vi "Get DSSS EVM.vi"(8 "error in (no error)":errorcluster, 11 "niDTS WLAN INSTR TX in":refnum<class "niDTS WLAN INSTR TX.lvclass">) -> (0 "error out":errorcluster, 2 "DSSS EVM":T1, 3 "niDTS WLAN INSTR TX out":refnum<class "niDTS WLAN INSTR TX.lvclass">)   [LabVIEW 2015, in "niDTS WLAN.lvlib" / "niDTS WLAN INSTR TX.lvclass"]
uses:
  niDTS WLAN INSTR TX.lvclass
  Tests/Tx Test/Includes/niDTS WLAN Tx Test INC DSSS MOD EVM Results.ctl
  Tests/DSSS Tx Test/Includes/Results/niDTS WLAN DSSS Tx RES EVM ALL.ctl
  Tests/DSSS Tx Test/Includes/Results/niDTS WLAN DSSS Tx RES EVM RMS.ctl
  niDTS WLAN INSTR TX.lvclass/niDTS WLAN INSTR TX.ctl
  RiviInstDriver/niRfsaWlan/Objects/niRfsaWlan.lvclass
  niDTS WLAN.lvlib
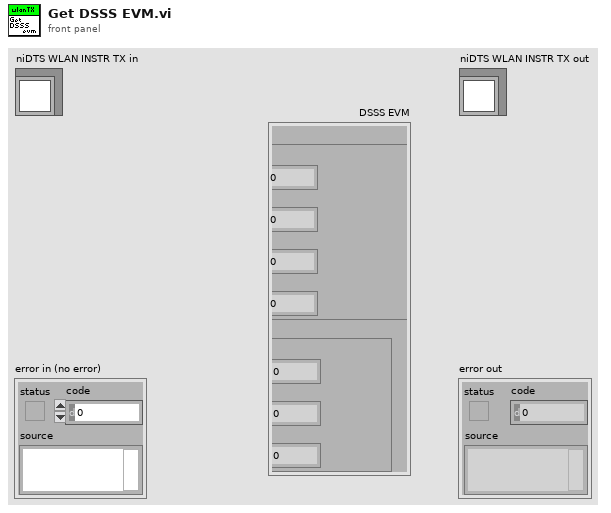
[diagram p1: front panel]
types:
  T1 = typedef "niDTS WLAN.lvlib/niDTS WLAN Tx Test INC DSSS MOD EVM Results.ctl" = cluster{"All":T2, "RMS":T3}
  T2 = typedef "niDTS WLAN.lvlib/niDTS WLAN DSSS Tx RES EVM ALL.ctl" = cluster{"Average RMS EVM (%)":dbl, "Max Peak EVM (%)":dbl, "Max Peak 11b EVM (%)":dbl, "New Max Peak 11b EVM (%)":dbl}
  T3 = typedef "niDTS WLAN.lvlib/niDTS WLAN DSSS Tx RES EVM RMS.ctl" = cluster{"Average RMS EVM (%)":dbl, "Max RMS EVM (%)":dbl, "Min RMS EVM (%)":dbl}
  T4 = cluster{"AverageRmsEvm":dbl, "MaxRmsEvm":dbl, "MinRmsEvm":dbl}
  T5 = cluster{"AverageRmsEvm":dbl, "MaxPeakEvm":dbl, "MaxPeak11bEvm":dbl, "NewMaxPeak11bEvm":dbl}
  T6 = typedef "niRfsaWlan.lvclass/niRfsaWlan INC Handle.ctl" = refnum<data-value>
  T7 = typedef "niDTS WLAN.lvlib/niDTS WLAN Tx Test INC Parameters.ctl" = cluster{"Standard":T8, "DSSS Data Rate (Mbps)":T9, "OFDM Data Rate (Mbps)":T10, "MCS Index":i32, "N spatial streams":i32, "Chains":bool[], "BandWidth (Hz)":T11, "Channel":i32, "Gard Interval":T12, "FEC Coding":T13, "Dut Tx Power":dbl, "16 symbols":bool, "payload length bytes":i32, "idle interval":dbl, "External Attenuation":dbl[], "Acquisition Parameters ":T14, "TXP Measurement Parameters":T15, "ModAcc Measurement Paramaters":T16, "ModAcc DSSS Paramaters":T17, "SEM Measurement Parameters":T19, "OBW Measurement Parameters":T20, "DSSS Power Ramp":T21, "Enable Traces":bool}
  T8 = typedef "niDTS WLAN.lvlib/niDTS WLAN INC Standard.ctl" = enum16{"802.11 b DSSS", "802.11 a/g OFDM", "802.11 n HT", "802.11 ac VHT"}
  T9 = typedef "niDTS WLAN.lvlib/niDTS WLAN INC DSSS Data Rate.ctl" = enum16{"1", "2", "5.5", "11"}
  T10 = typedef "niDTS WLAN.lvlib/niDTS WLAN INC OFDM Data Rate.ctl" = enum16{"6", "9", "12", "18", "24", "36", "48", "54"}
  T11 = typedef "niDTS WLAN.lvlib/niDTS WLAN INC CH BW.ctl" = enum16{"20 MHz", "40 MHz", "80 MHz", "160 MHz"}
  T12 = typedef "niDTS WLAN.lvlib/niDTS WLAN INC GI.ctl" = enum16{"LONG", "SHORT"}
  T13 = typedef "niDTS WLAN.lvlib/niDTS WLAN INC FEC Coding.ctl" = enum16{"BCC", "LDPC"}
  T14 = typedef "niDTS WLAN.lvlib/niDTS WLAN DUT INC Acquisition Parameters.ctl" = cluster{"Acquisition Length Mode":enum16{"AUTO", "MANUAL"}, "Acquisition Length (s)":dbl, "Auto Level":bool}
  T15 = typedef "niDTS WLAN.lvlib/niDTS WLAN INC TXP Measurement Parameters.ctl" = cluster{"TXP Power Enable":bool, "TXP Averages":i32}
  T16 = typedef "niDTS WLAN.lvlib/niDTS WLAN INC ModAcc Measurement Parameters.ctl" = cluster{"ModAcc Enable":bool, "Header Detection":enum16{"MANUAL", "FIRST", "ALL"}, "Averages":i32, "Amplitude Tracking":bool, "Channel Tracking":bool, "Time Tracking":bool, "Phase Tracking":enum16{"NONE", "STANDARD", "CSF", "INSTANT"}, "Clock Offset Est":bool, "Impairments Est":bool, "CFO Estimation":enum16{"PAMBLE", "PDATA"}}
  T17 = typedef "niDTS WLAN.lvlib/niDTS WLAN INC DSSS ModAcc Measurement Parameters.ctl" = cluster{"DC Offset Compensation":bool, "Equalization":bool, "Phase Tracking":bool, "Chip Start Location":i16, "Max Chips Used":i16, "Pulse Shaping FilterType":T18, "Pulse Shaping Filter Coefficient":dbl}
  T18 = typedef "niDTS WLAN.lvlib/niDTS WLAN INC Pulse Shaping Filter Type.ctl" = enum16{"NONE", "RCOSINE", "RRCOSINE", "GAUSSIAN"}
  T19 = typedef "niDTS WLAN.lvlib/niDTS WLAN INC SEM Measurement Parameters.ctl" = cluster{"SEM Enable":bool, "SEM Averages":i32, "Auto Span Enable":bool, "Frequency Span (Hz)":dbl, "Measurement Type":enum16{"Standard", "Legacy", "Custom"}, "Mask Frequencies (Hz)":dbl[], "Mask Power Offsets (dB)":dbl[]}
  T20 = typedef "niDTS WLAN.lvlib/niDTS WLAN INC OBW Measurement Parameters.ctl" = cluster{"OBW Enable":bool, "OBW Averages":i32}
  T21 = typedef "niDTS WLAN.lvlib/niDTS WLAN INC DSSS Power Ramp Parameters.ctl" = cluster{"Power Ramp Enable":bool, "Averages":i32, "Thresholds":cluster{"Up Low (%)":dbl, "Down Low (%)":dbl, "Up High (%)":dbl, "Down High (%)":dbl}}
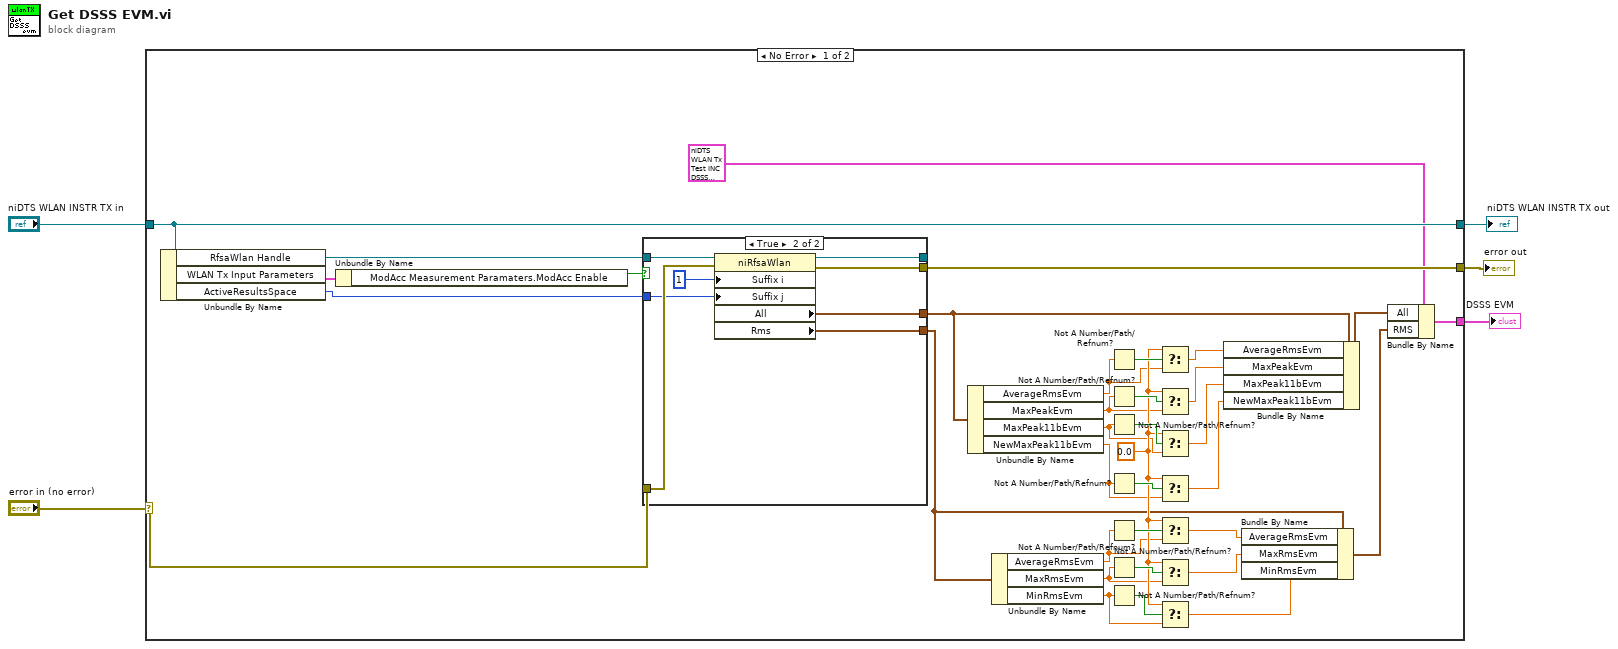
[diagram p0: block diagram]
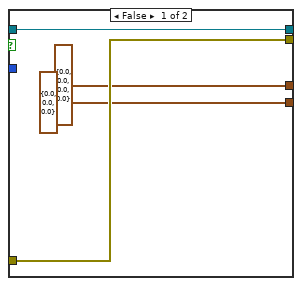
[diagram p2: hidden frame]
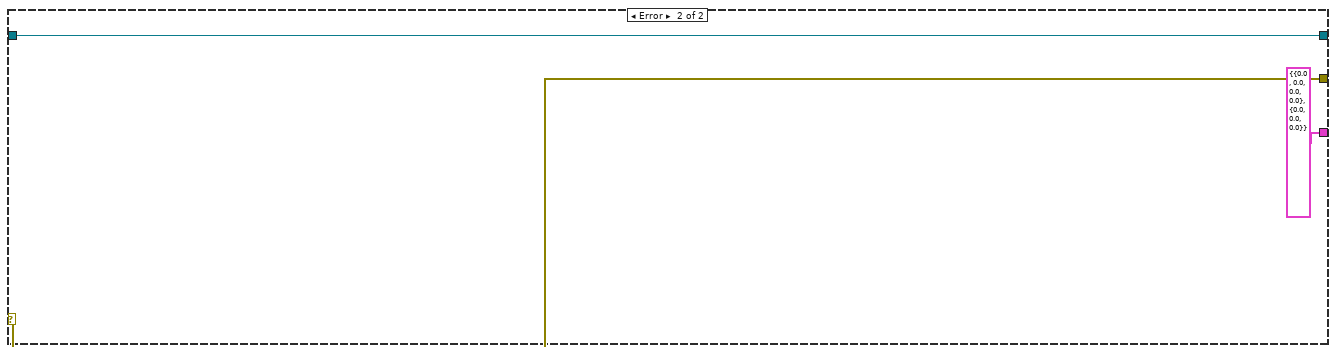
[diagram p3: hidden frame]
diagram:
  n1 = case shown="No Error" "error in (no error)" {
    selector: "error in (no error)" -> [w38 w55]
    tunnel: [w35 w55] -> w4
    tunnel: [w40 w54] -> w2
    tunnel: "niDTS WLAN INSTR TX in" -> [w40 w54]
    tunnel: [w34 T1 {"All"={"Average RMS EVM (%)"=0.0, "Max Peak EVM (%)"=0.0, "Max Peak 11b EVM (%)"=0.0, "New Max Peak 11b EVM (%)"=0.0}, "RMS"={"Average RMS EVM (%)"=0.0, "Max RMS EVM (%)"=0.0, "Min RMS EVM (%)"=0.0}} ("DSSS EVM")] -> w1
    frame No Error {
      w24 = 0.0
      n2 = Unbundle By Name(w40) -> ("RfsaWlan Handle"=w36:T6, "WLAN Tx Input Parameters"=w39:T7, "ActiveResultsSpace"=w33:u8)
      n3 = Unbundle By Name(w39) -> ("ModAcc Measurement Paramaters.ModAcc Enable"=w37:bool)
      n4 = case shown="True" w37 {
        tunnel: w38 -> [w43 w50]
        tunnel: w36 -> [w44 w51]
        tunnel: [w44 w49] -> _
        tunnel: [w43 w48] -> w35
        tunnel: w33 -> [_ w47]
        tunnel: [T5 {"AverageRmsEvm"=0.0, "MaxPeakEvm"=0.0, "MaxPeak11bEvm"=0.0, "NewMaxPeak11bEvm"=0.0} ("[ALL]") w46] -> w16
        tunnel: [T4 {"AverageRmsEvm"=0.0, "MaxRmsEvm"=0.0, "MinRmsEvm"=0.0} ("RMS") w45] -> w14
        frame False {
        }
        frame True {
          n5 = property class="niRfsaWlan"(reference=w51, error in=w50, "Suffix i"=1 ("Active Channel:Result Space"), "Suffix j"=w47) -> (reference out=w49:T6, error out=w48:errorcluster, "All"=w46:T5, "Rms"=w45:T4)
        }
      }
      n6 = Unbundle By Name(w16) -> ("AverageRmsEvm"=w23:dbl, "MaxPeakEvm"=w22:dbl, "MaxPeak11bEvm"=w21:dbl, "NewMaxPeak11bEvm"=w20:dbl)
      n7 = Unbundle By Name(w14) -> ("AverageRmsEvm"=w19:dbl, "MaxRmsEvm"=w18:dbl, "MinRmsEvm"=w17:dbl)
      n8 = Not A Number/Path/Refnum?(number/path/refnum=w23) -> (NaN/Path/Refnum?=w31:bool)
      n9 = Not A Number/Path/Refnum?(number/path/refnum=w22) -> (NaN/Path/Refnum?=w30:bool)
      n10 = Not A Number/Path/Refnum?(number/path/refnum=w21) -> (NaN/Path/Refnum?=w29:bool)
      n11 = Not A Number/Path/Refnum?(number/path/refnum=w20) -> (NaN/Path/Refnum?=w28:bool)
      n12 = Not A Number/Path/Refnum?(number/path/refnum=w19) -> (NaN/Path/Refnum?=w26:bool)
      n13 = Not A Number/Path/Refnum?(number/path/refnum=w18) -> (NaN/Path/Refnum?=w27:bool)
      n14 = Not A Number/Path/Refnum?(number/path/refnum=w17) -> (NaN/Path/Refnum?=w25:bool)
      n15 = Select(t=w24, s=w31, f=w23) -> (s? t:f=w7:dbl)
      n16 = Select(t=w24, s=w30, f=w22) -> (s? t:f=w8:dbl)
      n17 = Select(t=w24, s=w29, f=w21) -> (s? t:f=w9:dbl)
      n18 = Select(t=w24, s=w28, f=w20) -> (s? t:f=w10:dbl)
      n19 = Select(t=w24, s=w26, f=w19) -> (s? t:f=w12:dbl)
      n20 = Select(t=w24, s=w27, f=w18) -> (s? t:f=w13:dbl)
      n21 = Select(t=w24, s=w25, f=w17) -> (s? t:f=w11:dbl)
      n22 = Bundle By Name(cluster=w16, "AverageRmsEvm"=w7, "MaxPeakEvm"=w8, "MaxPeak11bEvm"=w9, "NewMaxPeak11bEvm"=w10) -> (w15:T5)
      n23 = Bundle By Name(cluster=w14, "AverageRmsEvm"=w12, "MaxRmsEvm"=w13, "MinRmsEvm"=w11) -> (w6:T4)
      n24 = Bundle By Name(cluster=T1 {"All"={"Average RMS EVM (%)"=0.0, "Max Peak EVM (%)"=0.0, "Max Peak 11b EVM (%)"=0.0, "New Max Peak 11b EVM (%)"=0.0}, "RMS"={"Average RMS EVM (%)"=0.0, "Max RMS EVM (%)"=0.0, "Min RMS EVM (%)"=0.0}} ("DSSS EVM"), "All"=w15, "RMS"=w6) -> (w34:T1)
    }
    frame Error {
    }
  }
  "error out" <- w4
  "niDTS WLAN INSTR TX out" <- w2
  "DSSS EVM" <- w1
